vi "Procedure Parameters (B).vi"(0 "LoadProcedure":refnum<k24>, 5 "Command Parameter":string(combo)="Start value", 7 "IntSet":i32, 9 "DoubleSet":dbl, 11 "error in (no error)":errorcluster) -> (15 "error out":errorcluster)   [LabVIEW 2011]
doc: "Changes the procedure parameters with constant values(basic version)."
uses:
  C:/Program Files/Metrohm Autolab/Autolab SDK 1.10/EcoChemie.Autolab.Sdk.dll
  EcoChemie.Autolab.Sdk.dll
  C:/Program Files/Metrohm Autolab/Autolab SDK 1.10/EcoChemie100.dll
  EcoChemie100.dll
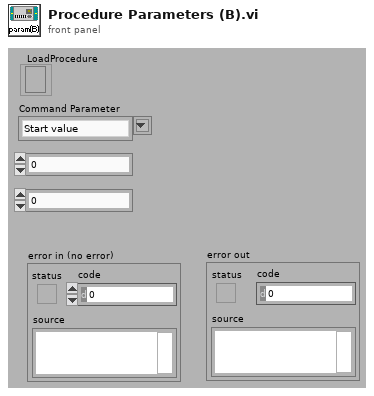
[diagram p1: front panel]
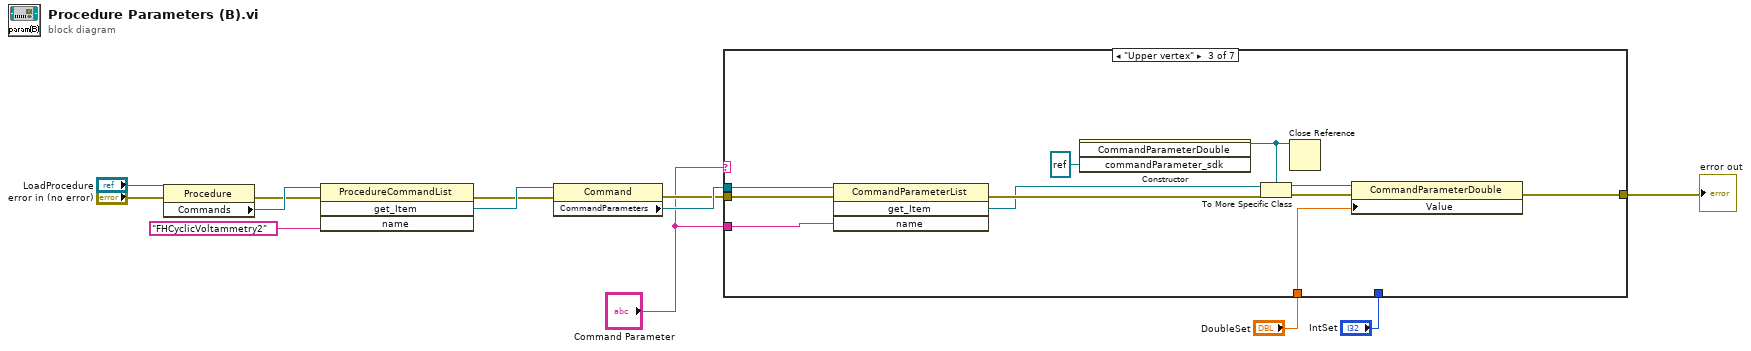
[diagram p0: block diagram]
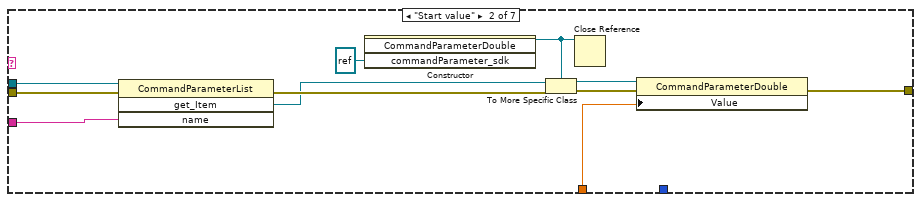
[diagram p3: hidden frame]
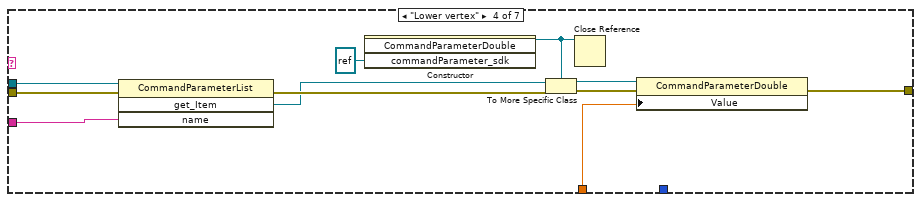
[diagram p4: hidden frame]
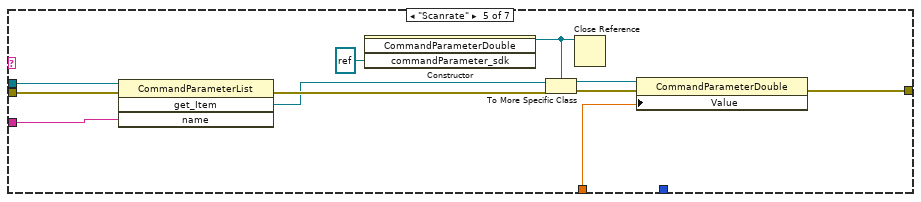
[diagram p5: hidden frame]
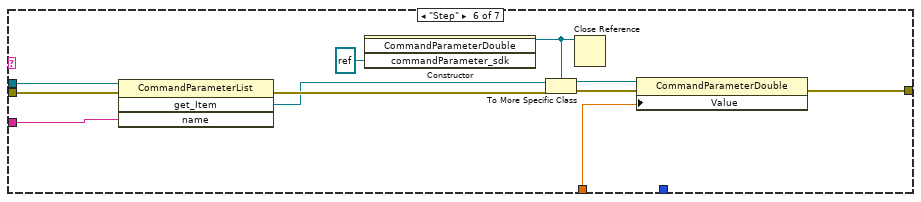
[diagram p6: hidden frame]
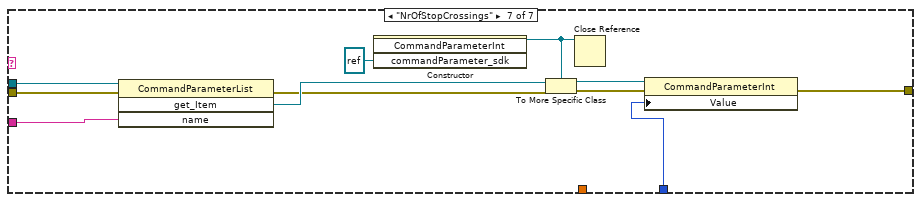
[diagram p7: hidden frame]
diagram:
  n1 = property class="Procedure"(reference="LoadProcedure", error in="error in (no error)") -> (error out=w9:errorcluster, "Commands"=w10:refnum<k24>)  [unwired: 1 out]
  n2 = invoke class="ProcedureCommandList" method="get_Item"(reference=w10, error in=w9, "name"="FHCyclicVoltammetry2" ("Command")) -> (error out=w11:errorcluster, "get_Item"=w12:refnum<k24>)  [unwired: 1 in, 2 out]
  n3 = property class="Command"(reference=w12, error in=w11) -> (error out=w7:errorcluster, "CommandParameters"=w8:refnum<k24>)  [unwired: 1 out]
  n4 = case shown="\"Upper vertex\"" "Command Parameter" {
    tunnel: w8 -> [_ w23 w33 w44 w55 w65 w77]
    tunnel: w7 -> [w14 w22 w32 w43 w54 w64 w76]
    tunnel: "Command Parameter" -> [_ w21 w31 w42 w53 w63 w75]
    tunnel: "DoubleSet" -> [_ w20 w30 w41 w52 w62 _]
    tunnel: "IntSet" -> [_ _ _ _ _ _ w74]
    tunnel: [w14 w19 w29 w40 w51 w61 w73] -> w2
    frame "False", Default {
    }
    frame "Start value" {
      n5 = invoke class="CommandParameterList" method="get_Item"(reference=w23, error in=w22, "name"=w21) -> (error out=w25:errorcluster, "get_Item"=w24:refnum<k24>)  [unwired: 1 in, 2 out]
      n6 = constructor class="CommandParameterDouble"("commandParameter_sdk"=refnum<k24> refnum) -> (reference out=w16:refnum<k24>)  [unwired: 3 in, 3 out]
      n7 = To More Specific Class(target class=w16, reference=w24, error in=w25) -> (specific class reference=w18:refnum<k24>, error out=w17:errorcluster)
      n8 = Close Reference(reference=w16) -> ()  [unwired: 1 in, 1 out]
      n9 = property class="CommandParameterDouble"(reference=w18, error in=w17, "Value"=w20) -> (error out=w19:errorcluster)  [unwired: 1 out]
    }
    frame "Upper vertex" {
      n10 = invoke class="CommandParameterList" method="get_Item"(reference=w33, error in=w32, "name"=w31) -> (error out=w36:errorcluster, "get_Item"=w35:refnum<k24>)  [unwired: 1 in, 2 out]
      n11 = constructor class="CommandParameterDouble"("commandParameter_sdk"=refnum<k24> refnum) -> (reference out=w27:refnum<k24>)  [unwired: 3 in, 3 out]
      n12 = To More Specific Class(target class=w27, reference=w35, error in=w36) -> (specific class reference=w34:refnum<k24>, error out=w28:errorcluster)
      n13 = Close Reference(reference=w27) -> ()  [unwired: 1 in, 1 out]
      n14 = property class="CommandParameterDouble"(reference=w34, error in=w28, "Value"=w30) -> (error out=w29:errorcluster)  [unwired: 1 out]
    }
    frame "Lower vertex" {
      n15 = invoke class="CommandParameterList" method="get_Item"(reference=w44, error in=w43, "name"=w42) -> (error out=w47:errorcluster, "get_Item"=w46:refnum<k24>)  [unwired: 1 in, 2 out]
      n16 = constructor class="CommandParameterDouble"("commandParameter_sdk"=refnum<k24> refnum) -> (reference out=w38:refnum<k24>)  [unwired: 3 in, 3 out]
      n17 = To More Specific Class(target class=w38, reference=w46, error in=w47) -> (specific class reference=w45:refnum<k24>, error out=w39:errorcluster)
      n18 = Close Reference(reference=w38) -> ()  [unwired: 1 in, 1 out]
      n19 = property class="CommandParameterDouble"(reference=w45, error in=w39, "Value"=w41) -> (error out=w40:errorcluster)  [unwired: 1 out]
    }
    frame "Scanrate" {
      n20 = invoke class="CommandParameterList" method="get_Item"(reference=w55, error in=w54, "name"=w53) -> (error out=w58:errorcluster, "get_Item"=w57:refnum<k24>)  [unwired: 1 in, 2 out]
      n21 = constructor class="CommandParameterDouble"("commandParameter_sdk"=refnum<k24> refnum) -> (reference out=w49:refnum<k24>)  [unwired: 3 in, 3 out]
      n22 = To More Specific Class(target class=w49, reference=w57, error in=w58) -> (specific class reference=w56:refnum<k24>, error out=w50:errorcluster)
      n23 = Close Reference(reference=w49) -> ()  [unwired: 1 in, 1 out]
      n24 = property class="CommandParameterDouble"(reference=w56, error in=w50, "Value"=w52) -> (error out=w51:errorcluster)  [unwired: 1 out]
    }
    frame "Step" {
      n25 = invoke class="CommandParameterList" method="get_Item"(reference=w65, error in=w64, "name"=w63) -> (error out=w69:errorcluster, "get_Item"=w68:refnum<k24>)  [unwired: 1 in, 2 out]
      n26 = constructor class="CommandParameterDouble"("commandParameter_sdk"=refnum<k24> refnum) -> (reference out=w60:refnum<k24>)  [unwired: 3 in, 3 out]
      n27 = To More Specific Class(target class=w60, reference=w68, error in=w69) -> (specific class reference=w67:refnum<k24>, error out=w66:errorcluster)
      n28 = Close Reference(reference=w60) -> ()  [unwired: 1 in, 1 out]
      n29 = property class="CommandParameterDouble"(reference=w67, error in=w66, "Value"=w62) -> (error out=w61:errorcluster)  [unwired: 1 out]
    }
    frame "NrOfStopCrossings" {
      n30 = invoke class="CommandParameterList" method="get_Item"(reference=w77, error in=w76, "name"=w75) -> (error out=w78:errorcluster, "get_Item"=w79:refnum<k24>)  [unwired: 1 in, 2 out]
      n31 = constructor class="CommandParameterInt"("commandParameter_sdk"=refnum<k24> refnum) -> (reference out=w71:refnum<k24>)  [unwired: 3 in, 3 out]
      n32 = To More Specific Class(target class=w71, reference=w79, error in=w78) -> (specific class reference=w80:refnum<k24>, error out=w72:errorcluster)
      n33 = Close Reference(reference=w71) -> ()  [unwired: 1 in, 1 out]
      n34 = property class="CommandParameterInt"(reference=w80, error in=w72, "Value"=w74) -> (error out=w73:errorcluster)  [unwired: 1 out]
    }
  }
  "error out" <- w2
